vi "Monitor Temp.vi"(8 "error in (no error)":errorcluster, 10 "Address (0)":i32, 11 "VISA resource name":refnum<visa-resource-name>) -> (0 "error out":errorcluster, 1 "temp setpoint":dbl, 2 "measured temp":dbl, 3 "VISA resource name out":refnum<visa-resource-name>, 4 "lower limit alarm":dbl, 5 "upper limit alarm":dbl)   [LabVIEW 2016, in "Environment Chamber.lvlib" / "Climatic Chamber.lvlib"]
doc: "<b>Temperature setting monitor</B>\n\nMonitors information related to the temperature."
uses:
  Climatic Chamber.lvlib
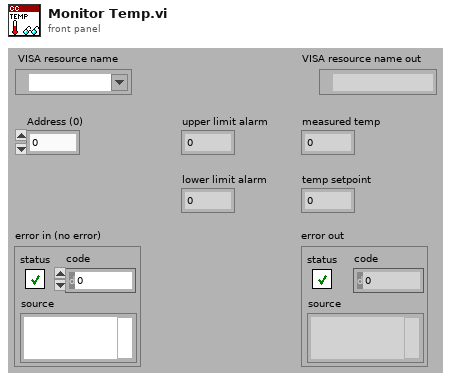
[diagram p1: front panel]
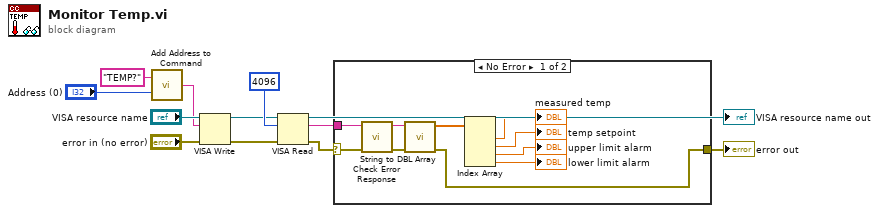
[diagram p0: block diagram]
diagram:
  n1 = call "Add Address to Command.vi"("Address (0)"="Address (0)", "Command"="TEMP?") -> ("Command OUT"=w4:string)
  n2 = VISA Write(VISA resource name="VISA resource name", write buffer=w4, error in (no error)="error in (no error)") -> (VISA resource name out=w9:refnum<visa-resource-name>, error out=w8:errorcluster)  [unwired: 1 out]
  n3 = VISA Read(VISA resource name=w9, byte count=u32 4096, error in (no error)=w8) -> (VISA resource name out=→"VISA resource name out":refnum<visa-resource-name>, read buffer=w2:string, error out=w3:errorcluster)  [unwired: 1 out]
  n4 = case shown="No Error" w3 {
    selector: w3 -> [w15 w23]
    tunnel: w2 -> [w17 _]
    tunnel: [w13 w23] -> w1
    frame No Error {
      n5 = call "Check Error Response.vi"("error in (no error)"=w15, "read String"=w17) -> ("error out"=w14:errorcluster, "String out"=w16:string)  [unwired: 7 in, 1 out]
      n6 = call "String to DBL Array.vi"("error in (no error)"=w14, "String received"=w16) -> ("error out"=w13:errorcluster, "Array Data"=w22:dbl[])  [unwired: 8 in]
      n7 = Index Array(array=w22) -> (element #1=→"measured temp":dbl, element #2=→"temp setpoint":dbl, element #3=→"upper limit alarm":dbl, element #4=→"lower limit alarm":dbl)  [unwired: 4 in]
    }
    frame Error {
    }
  }
  "error out" <- w1
